vi "Utility-Create Base path and-or filename.vi"(10 "filename":string, 11 "Directory Name":T1=enum."config") -> (2 "File name and path":path)   [LabVIEW 2014]
uses:
  TypeDef - Directory Structures.ctl
  <vilib>/Utility/sysdir.llb/System Directory Type.ctl
  Utilities/Global - Demo Mode Flags.vi
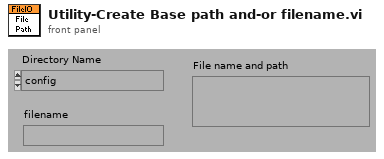
[diagram p1: front panel]
types:
  T1 = typedef "TypeDef - Directory Structures.ctl" = enum16{"Project", "config", "testconfig", "raw data"}
  T2 = typedef "System Directory Type.ctl" = i32
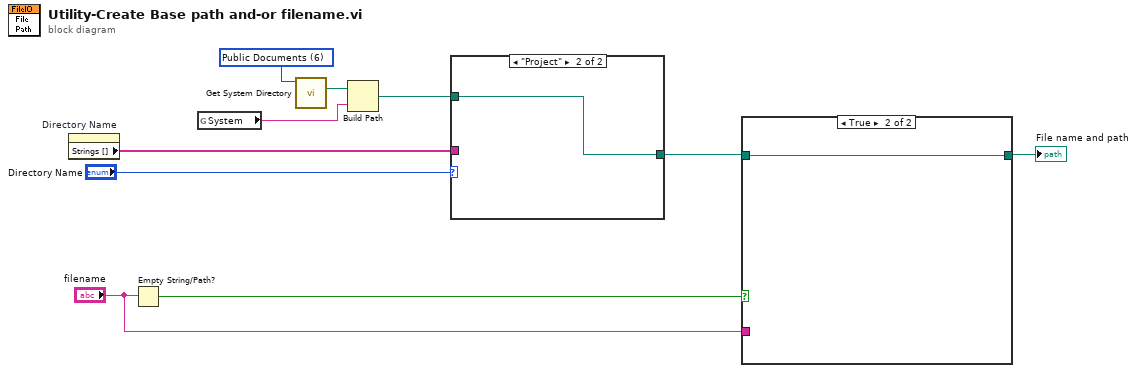
[diagram p0: block diagram]
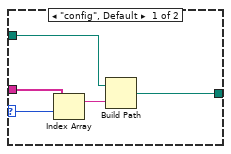
[diagram p2: hidden frame]
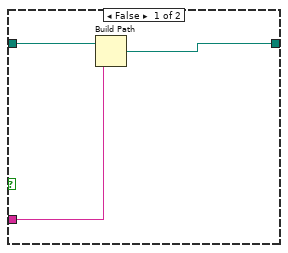
[diagram p3: hidden frame]
diagram:
  w4 = T2 6 items=["User Home"=0, "User Desktop"=1, "User Documents"=2, "User Application Data"=3, "User Preferences"=4, "User Temporary"=5, "Public Documents"=6, "Public Application Data"=7, "Public Preferences"=8, "Public Cache"=13, "System Core Libraries"=9, "System Installed Libraries"=10, "Application Files"=11, "Boot Volume Root"=12] ("system directory type")
  n1 = property on="Directory Name" class="Enum (strict)"() -> ("Strings []"=w10:string[])  [unwired: 2 in, 2 out]
  n2 = Empty String/Path?(string/path="filename") -> (empty?=w5:bool)
  n3 = global read "Global - Demo Mode Flags.vi" "System"() -> (w1:string)
  n4 = call <vilib>:"Get System Directory.vi"("system directory type"=w4) -> ("system directory"=w3:path)  [unwired: 10 in]
  n5 = Build Path(base path=w3, name or relative path=w1) -> (appended path=w2:path)
  n6 = case shown="\"Project\"" "Directory Name" {
    selector: "Directory Name" -> [w12 _]
    tunnel: w10 -> [w15 _]
    tunnel: [w13 w16] -> w8
    tunnel: w2 -> [w11 w16]
    frame "config", Default {
      n7 = Index Array(array=w15, index=w12) -> (element=w14:string)
      n8 = Build Path(base path=w11, name or relative path=w14) -> (appended path=w13:path)
    }
    frame "Project" {
    }
  }
  n9 = case shown="True" w5 {
    tunnel: [w19 w20] -> w7
    tunnel: w8 -> [w18 w20]
    tunnel: "filename" -> [w17 _]
    frame False {
      n10 = Build Path(base path=w18, name or relative path=w17) -> (appended path=w19:path)
    }
    frame True {
    }
  }
  "File name and path" <- w7
